vi "move_to.vi"(6 "Wait until done":bool=TRUE, 8 "Error in":errorcluster, 9 "Axis names":string[](array[string])=["X", "Y", "Z", "Rx", "Ry", "Rz"], 10 "Axis positions":dbl[](array[numeric]), 11 "Mode":enum16{"Absolute axis", "Relative axis", "Pose"}(ring)) -> (0 "Error out":errorcluster)   [LabVIEW 2013]
uses:
  server/motion_command.ctl
panel:
  # "Move the stage to the specified position.  If \"Wait until done\" is true, then wait until the motion has completed before returning.  The axes to control are determined by the \"Axis names\" vector, allowing a subset of axes to be controlled.  Translation is in mm and angles in degrees.  \"Mode\" determines the interpretation of the \"Axis positions\".   The \"End transform\" and \"Home position\" (set by other VIs) can be used to transform the positions into a different coordinate system.\n\nIn \"Absolute axis\" mode the positions are absolute positions for the stage axes.   \"Home position\" is added to the axis positions and \"End transform\" is ignored.\n \nIn \"Relative axis\" mode the positions are offsets relative to the current stage position.  \"Home position\" and \"End transform\" have no effect.\n\nIn \"Pose\" mode, the positions are interpreted as a pose using ZYX Euler angles.  The \"End transform\" can be understood as the null pose of an end-effector (in stage coordinates.)   \"Home position\" is an additional 6DOF transform applied to the pose, creating an offset in the stage coordinates."
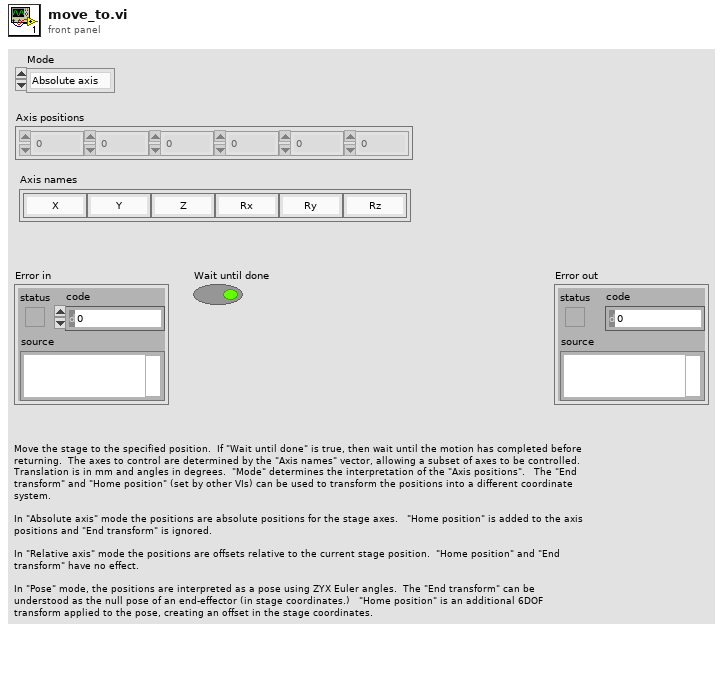
[diagram p1: front panel]
types:
  T1 = typedef "motion_status.ctl" = cluster{"Axis names":string[], "Axis positions":dbl[], "Pose":dbl[], "Timestamp":u32, "Ready":bool, "Stopped":bool}
  T2 = typedef "motion_command.ctl" = cluster{"Position":dbl[], "Axis enable":bool[], "Mode":enum16{"Absolute axis", "Relative axis", "Pose"}, "Timestamp":u32}
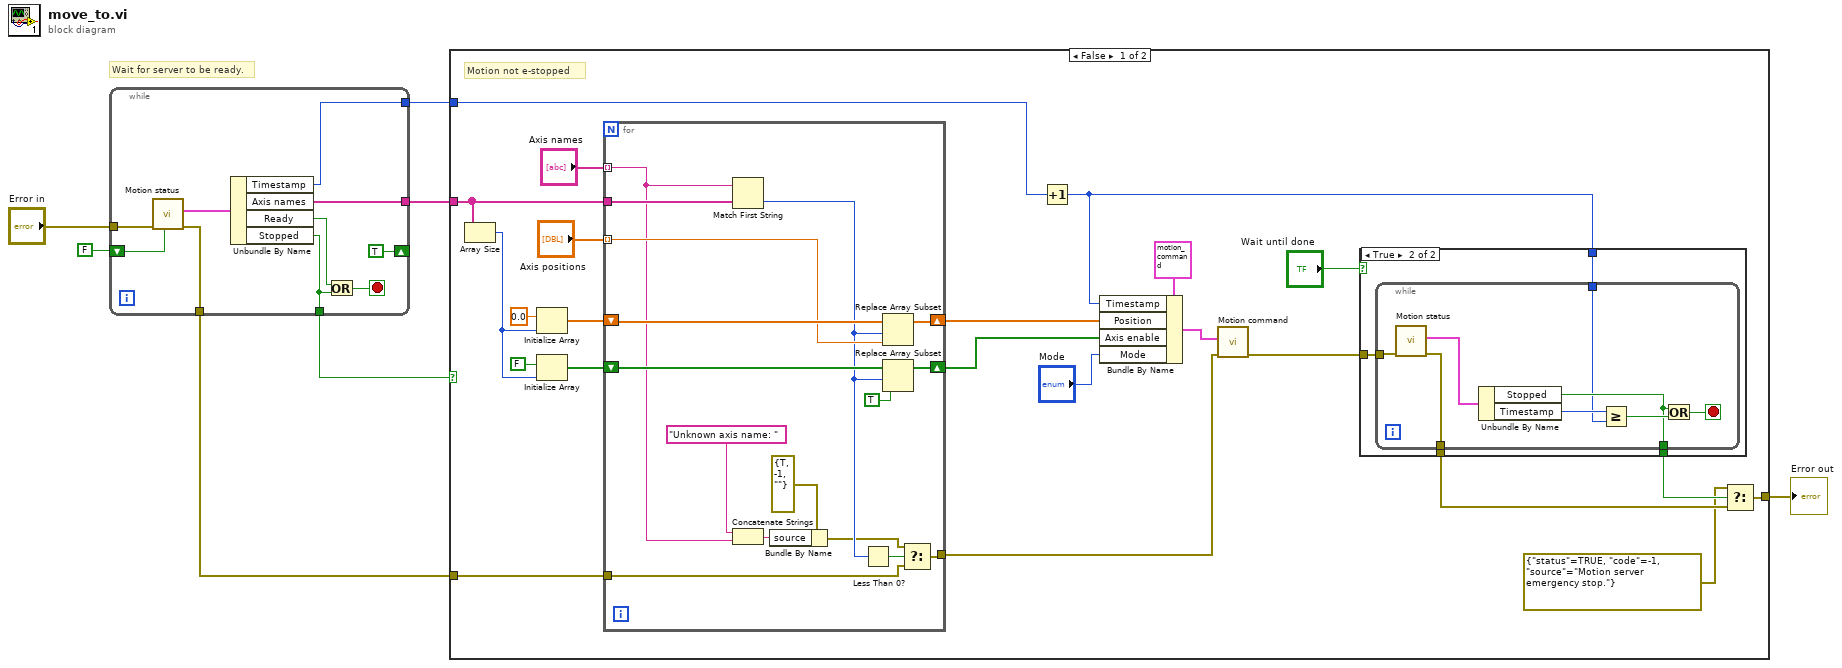
[diagram p0: block diagram]
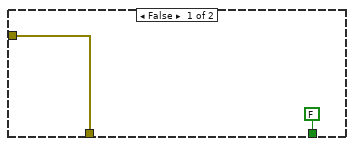
[diagram p2: hidden frame]
diagram:
  # "Wait for server to be ready."
  n1 = while {
    shift-right: [TRUE] -> _
    shift-left: FALSE -> [w17]
    tunnel: [w14] -> w6
    tunnel: "Error in" -> [w13]
    tunnel: [w10] -> w4
    tunnel: [w9] -> w2
    tunnel: [w8] -> w1
    stop <- w11 stop-if-true
    n2 = call "Motion status.vi"("Wait for updated value (F)"=w17, "error in"=w13) -> ("error out"=w10:errorcluster, "Motion status"=w15:T1)  [unwired: 4 in, 4 out]
    n3 = Unbundle By Name(w15) -> ("Timestamp"=w8:u32, "Axis names"=w14:string[], "Ready"=w12:bool, "Stopped"=w9:bool)
    n4 = Or(x=w12, y=w9) -> (x .or. y?=w11:bool)
  }
  n5 = case shown="False" w2 {
    tunnel: w6 -> [w40 _]
    tunnel: w4 -> [w24 w71]
    tunnel: [w21 w71] -> w3
    tunnel: w1 -> [w20 _]
    frame False {
      # "Motion not e-stopped"
      n6 = Array Size(array=w40) -> (size(s)=w33:i32)
      n7 = Initialize Array(0.0 ("element"), w33) -> (w36:dbl[])
      n8 = Initialize Array(FALSE ("Wait until done"), w33) -> (w32:bool[])
      n9 = for {
        tunnel: "Axis names" -> [w60] mode=indexing
        tunnel: "Axis positions" -> [w67] mode=indexing
        tunnel: w40 -> [w70]
        shift-right: [w64] -> w30
        shift-left: w36 -> [w69]
        shift-right: [w65] -> w29
        shift-left: w32 -> [w68]
        tunnel: [w61] -> w26
        tunnel: w24 -> [w55]
        n10 = Match First String(2:w70, 3:w60) -> (0:w63:i32)  [unwired: 1 out]
        n11 = Concatenate Strings("Unknown axis name: " ("string"), w60) -> (w58:string)
        n12 = Bundle By Name(cluster=errorcluster {"status"=TRUE, "code"=-1, "source"=""} ("Error in"), "source"=w58) -> (w56:errorcluster)
        n13 = Less Than 0?(x=w63) -> (x < 0?=w62:bool)
        n14 = Replace Array Subset(array=w69, new element=w67, index=w63) -> (w64:dbl[])
        n15 = Replace Array Subset(array=w68, new element=TRUE ("Wait until done"), index=w63) -> (w65:bool[])
        n16 = Select(t=w56, s=w62, f=w55) -> (s? t:f=w61:errorcluster)
      }
      n17 = Increment(x=w20) -> (x+1=w19:u32)
      n18 = Bundle By Name(cluster=T2 {"Position"=[0.0, 0.0], "Axis enable"=[TRUE, TRUE], "Mode"=enum."Absolute axis", "Timestamp"=0} ("Motion command"), "Timestamp"=w19, "Position"=w30, "Axis enable"=w29, "Mode"="Mode") -> (w27:T2)
      n19 = call "Motion command.vi"("error in"=w26, "Command"=w27) -> ("error out"=w39:errorcluster)  [unwired: 9 in]
      n20 = case shown="True" "Wait until done" {
        tunnel: w39 -> [w42 w46]
        tunnel: [w42 w45] -> w23
        tunnel: [FALSE ("Stopped") w44] -> w22
        tunnel: w19 -> [_ w43]
        frame False {
        }
        frame True {
          n21 = while {
            tunnel: w46 -> [w52]
            tunnel: [w49] -> w45
            tunnel: [w48] -> w44
            tunnel: w43 -> [w47]
            stop <- w51 stop-if-true
            n22 = call "Motion status.vi"("error in"=w52) -> ("error out"=w49:errorcluster, "Motion status"=w54:T1)  [unwired: 5 in, 4 out]
            n23 = Unbundle By Name(w54) -> ("Stopped"=w48:bool, "Timestamp"=w53:u32)
            n24 = Greater Or Equal?(x=w53, y=w47) -> (x >= y?=w50:bool)
            n25 = Or(x=w48, y=w50) -> (x .or. y?=w51:bool)
          }
        }
      }
      n26 = Select(t=errorcluster {"status"=TRUE, "code"=-1, "source"="Motion server emergency stop."} ("error out"), s=w22, f=w23) -> (s? t:f=w21:errorcluster)
    }
    frame True {
      # "E-stop abort"
    }
  }
  "Error out" <- w3
